vi "KE622x -- Get Service Request Event Enable Reg State.vi"(0 "VISA Resource In":refnum<visa-resource-name>, 1 "Error Query (T)?":bool=TRUE, 11 "error in (no error)":errorcluster) -> (4 "VISA Resource Out (dupl)":refnum<visa-resource-name>, 8 "KE622x Service Request Enable Reg State":T1, 15 "error out":errorcluster)   [LabVIEW 2019, in "Keithley 622x.lvlib"]
doc: "Returns the bits in the 'Service Request Enable' register of the Status Model. Note that only the used (named) bits are returned."
uses:
  Keithley 622x.lvlib
  Typedefs/KE622x -- Service Request Enable Reg State.ctl
panel:
  out "Reg Num (dec)":u16 format="%0d"
  out "Reg Num (binary)":u16 format="%016b"
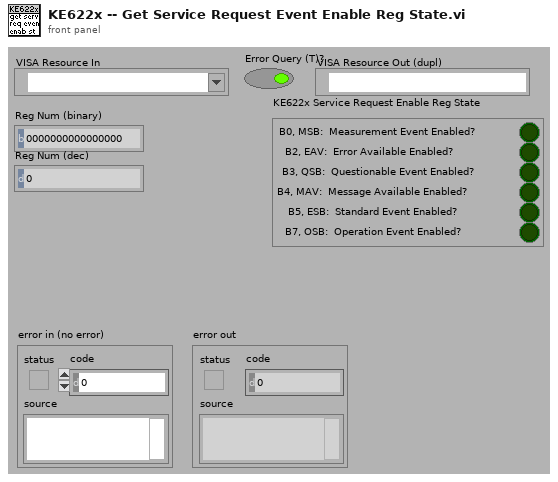
[diagram p1: front panel]
types:
  T1 = typedef "Keithley 622x.lvlib/KE622x -- Service Request Enable Reg State.ctl" = cluster{"B0, MSB:  Measurement Event Enabled?":bool, "B2, EAV:  Error Available Enabled?":bool, "B3, QSB:  Questionable Event Enabled?":bool, "B4, MAV:  Message Available Enabled?":bool, "B5, ESB:  Standard Event Enabled?":bool, "B7, OSB:  Operation Event Enabled?":bool}
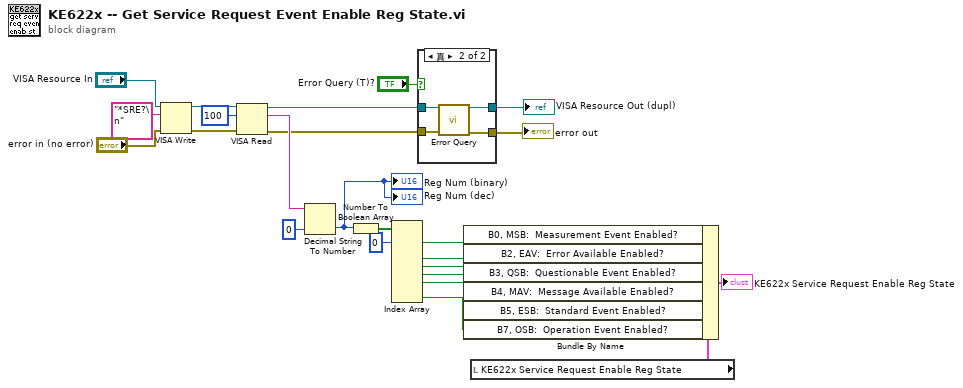
[diagram p0: block diagram]
diagram:
  n1 = VISA Write(VISA resource name="VISA Resource In", write buffer="*SRE?\n", error in (no error)="error in (no error)") -> (VISA resource name out=w21:refnum<visa-resource-name>, error out=w20:errorcluster)  [unwired: 1 out]
  n2 = VISA Read(VISA resource name=w21, byte count=u32 100, error in (no error)=w20) -> (VISA resource name out=w4:refnum<visa-resource-name>, read buffer=w18:string, error out=w3:errorcluster)  [unwired: 1 out]
  n3 = Decimal String To Number(string=w18, default (0L)=u16 0 ("default (0 I32)")) -> (number=w11:u16)  [unwired: 2 out]
  "Reg Num (binary)" <- w11
  "Reg Num (dec)" <- w11
  n4 = Number To Boolean Array(number=w11) -> (Boolean array=w16:bool[])
  n5 = Index Array(array=w16, index #1=0 ("index")) -> (element #1=w13:bool, element #3=w10:bool, element #4=w9:bool, element #5=w8:bool, element #6=w7:bool, element #8=w6:bool)  [unwired: 7 in, 2 out]
  n6 = case shown="真" "Error Query (T)?" {
    tunnel: w3 -> [w25 w30]
    tunnel: w4 -> [w26 w29]
    tunnel: [w25 w28] -> w1
    tunnel: [w26 w27] -> w2
    frame False {
    }
    frame True {
      n7 = call "Error Query.vi"("VISA Resource In"=w29, "error in (no error)"=w30) -> ("VISA Resource Out (dupl)"=w27:refnum<visa-resource-name>, "error out"=w28:errorcluster)  [unwired: 10 in, 2 out]
    }
  }
  "VISA Resource Out (dupl)" <- w2
  "error out" <- w1
  n8 = local read "KE622x Service Request Enable Reg State"() -> (w14:T1)
  n9 = Bundle By Name(cluster=w14, "B0, MSB:  Measurement Event Enabled?"=w13, "B2, EAV:  Error Available Enabled?"=w10, "B3, QSB:  Questionable Event Enabled?"=w9, "B4, MAV:  Message Available Enabled?"=w8, "B5, ESB:  Standard Event Enabled?"=w7, "B7, OSB:  Operation Event Enabled?"=w6) -> (→"KE622x Service Request Enable Reg State":T1)
